vi "Calculadora 1.vi"() -> ()   [LabVIEW 2019]
uses:
  <vilib>/gmath/NI_Gmath.lvlib
panel:
  in  "1/x\nx!":bool
  in  "Ln":bool
  in  "ans":bool
  in  "Pi\ne":bool
  in  "rt^x":bool
  in  "Ship":bool
  in  "e^x":bool
  in  "x^2\nsqrt":bool
  in  "Tanh":bool
  in  "Cosh":bool
  in  "Senh":bool
  in  "Logx":bool
  in  "Tan\nTan^-1":bool
  in  "Cos \nCos^-1":bool
  in  "Sen \nSen^-1":bool
  out "PANTALLA":string
  in  "AC":bool
  in  "C":bool
  in  "+":bool
  in  "=":bool
  in  "0":bool
  in  "/":bool
  in  "9":bool
  in  "8":bool
  in  "7":bool
  in  "X":bool
  in  "6":bool
  in  "5":bool
  in  "4":bool
  in  "-":bool
  in  "3":bool
  in  "2":bool
  in  "1":bool
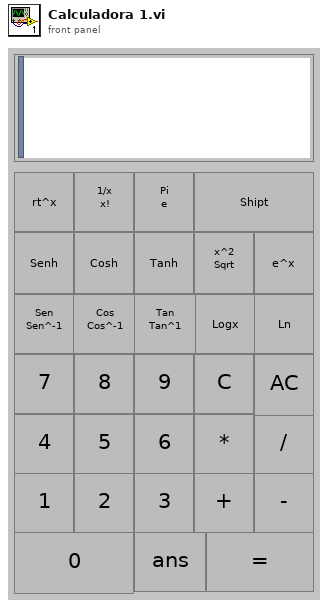
[diagram p1: front panel]
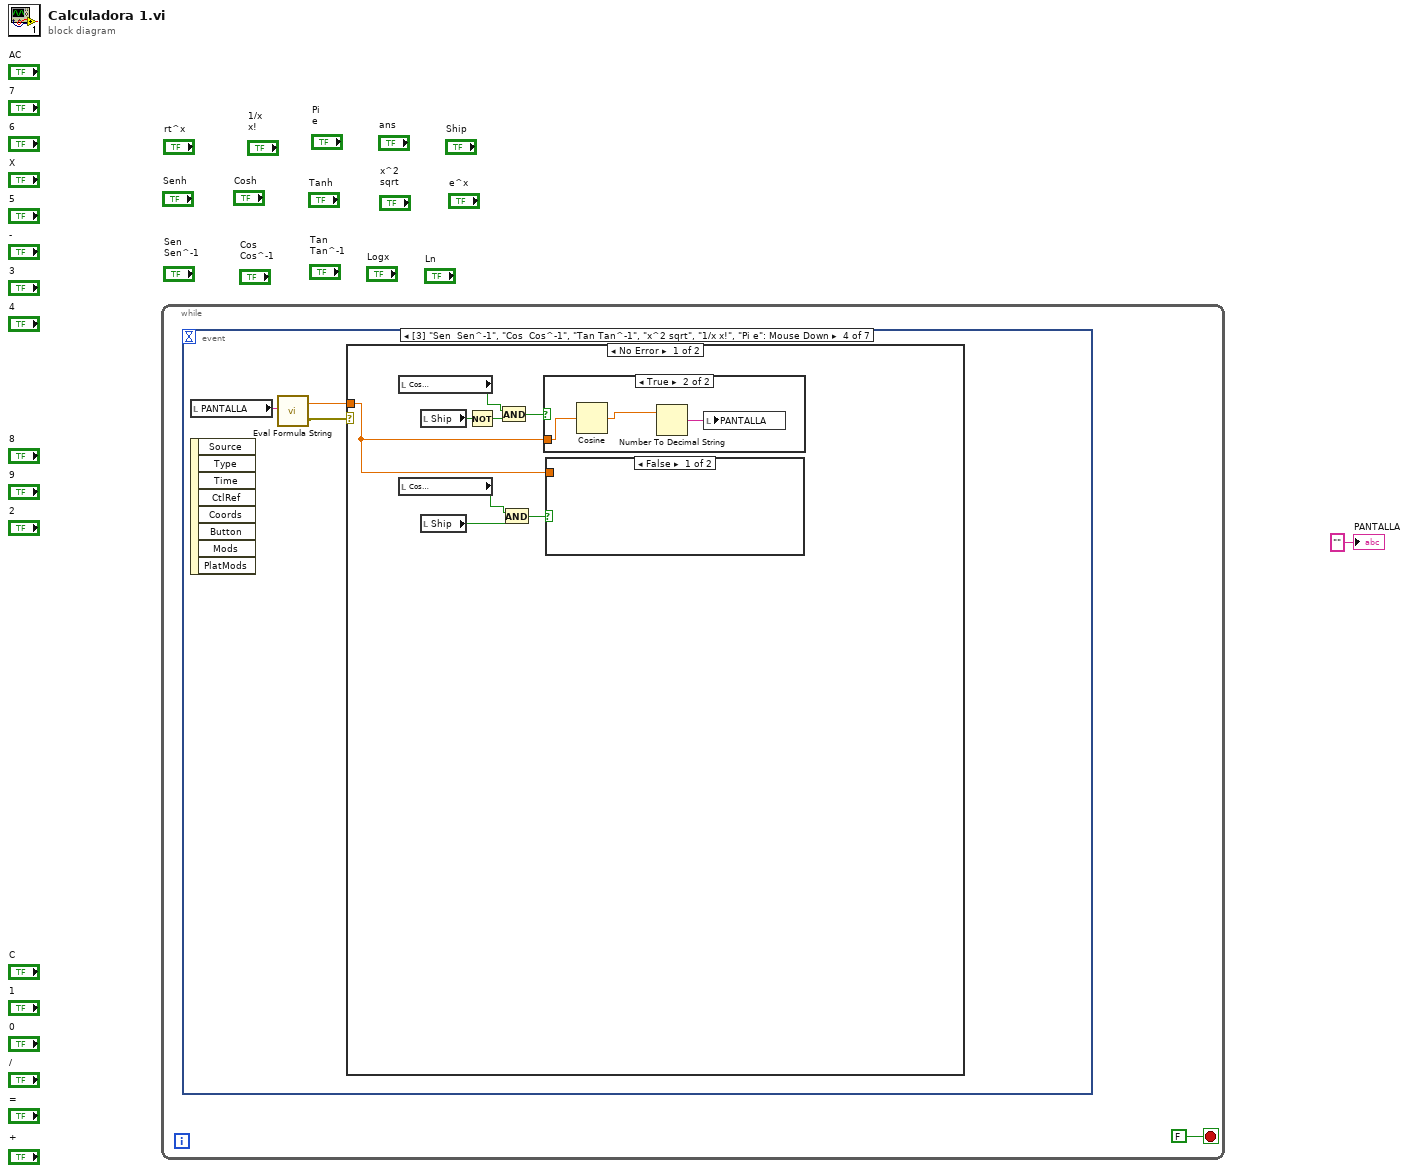
[diagram p0: block diagram]
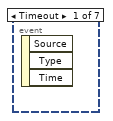
[diagram p2: hidden frame]
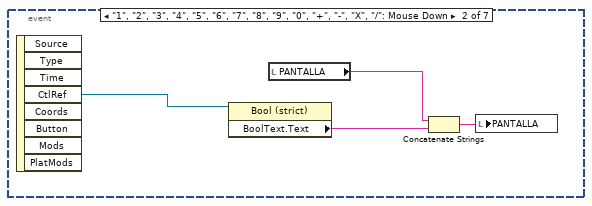
[diagram p3: hidden frame]
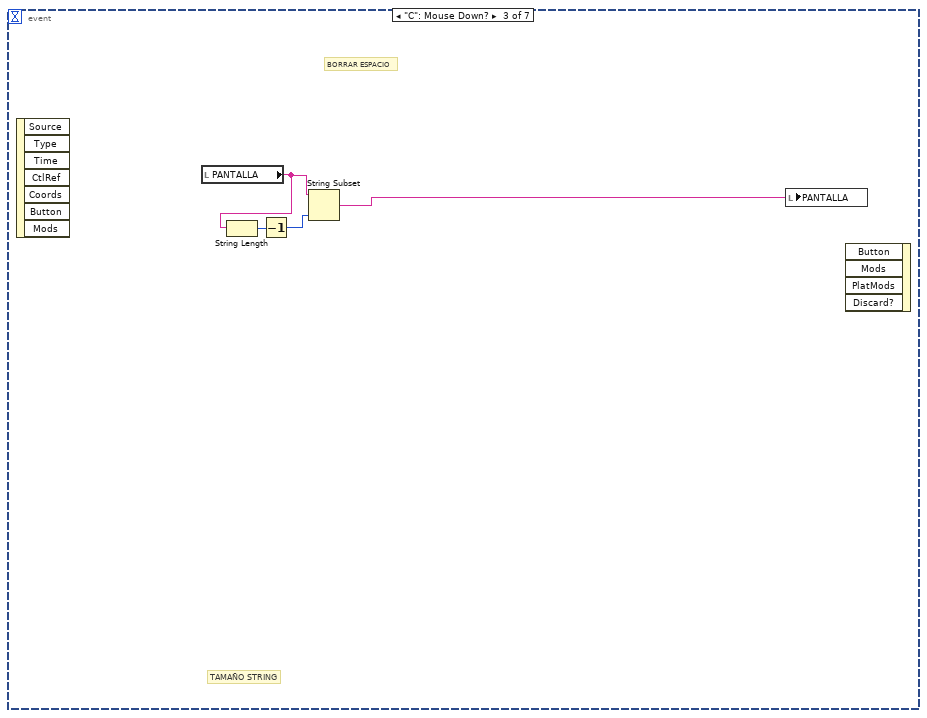
[diagram p4: hidden frame]
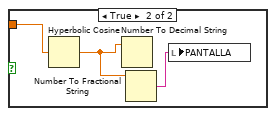
[diagram p6: hidden frame]
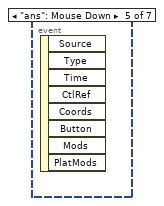
[diagram p8: hidden frame]
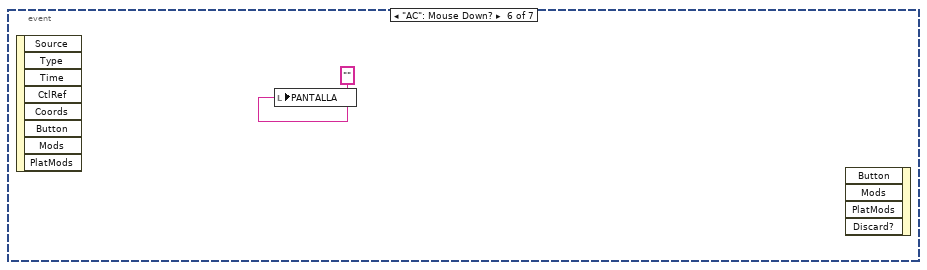
[diagram p9: hidden frame]
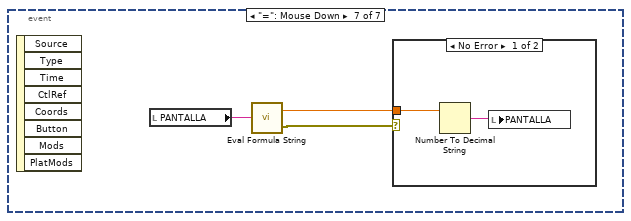
[diagram p10: hidden frame]
diagram:
  n1 = while {
    stop <- FALSE stop-if-true
    n2 = event shown="[3] \"Sen  Sen^-1\", \"Cos  Cos^-1\", \"Tan Tan^-1\", \"x^2 sqrt\", \"1/x x!\", \"Pi e\": Mouse Down" {
      selector: _ -> [_ _ _ _ _ _ _]
      dyn-events: _ -> [_ _ _ _ _ _ _]
      timeout: _ -> [_ _ _ _ _ _ _]
      event Timeout {
        n3 = event-data() -> ()  [unwired: 1 in, 3 out]
      }
      event "1", "2", "3", "4", "5", "6", "7", "8", "9", "0", "+", "-", "X", "/": Mouse Down {
        n4 = event-data() -> ("CtlRef"=w5:refnum<vi>)  [unwired: 1 in, 7 out]
        n5 = property class="Bool (strict)"(reference=w5) -> ("BoolText.Text"=w6:string)  [unwired: 1 in, 2 out]
        n6 = local read "PANTALLA"() -> (w4:string)
        n7 = Concatenate Strings(w4, w6) -> (w3:string)
        n8 = local write "PANTALLA"(w3) -> ()
      }
      event "C": Mouse Down? {
        # "BORRAR ESPACIO"
        # "TAMAÑO STRING"
        n9 = event-data() -> ()  [unwired: 1 in, 7 out]
        n10 = local read "PANTALLA"() -> (w10:string)
        n11 = String Length(string=w10) -> (length=w9:i32)
        n12 = Decrement(x=w9) -> (x-1=w8:i32)
        n13 = String Subset(string=w10, length (rest)=w8) -> (substring=w7:string)  [unwired: 1 in]
        n14 = local write "PANTALLA"(w7) -> ()
        n15 = event-data() -> ()  [unwired: 5 in, 1 out]
      }
      event "Sen \nSen^-1", "Cos \nCos^-1", "Tan\nTan^-1", "x^2\nsqrt", "1/x\nx!", "Pi\ne": Mouse Down {
        n16 = local read "PANTALLA"() -> (w11:string)
        n17 = event-data() -> ()  [unwired: 1 in, 8 out]
        n18 = call <vilib>:"Eval Formula String.vi"("formula"=w11) -> ("error out"=w13:errorcluster, "y value"=w12:dbl)  [unwired: 1 in]
        n19 = case shown="No Error" w13 {
          tunnel: w12 -> [w16 _]
          frame No Error {
            n20 = local read "Cos \nCos^-1"() -> (w18:bool)
            n21 = local read "Cos \nCos^-1"() -> (w19:bool)
            n22 = local read "Ship"() -> (w14:bool)
            n23 = local read "Ship"() -> (w20:bool)
            n24 = Not(x=w14) -> (.not. x?=w15:bool)
            n25 = And(x=w18, y=w15) -> (x .and. y?=w17:bool)
            n26 = And(x=w19, y=w20) -> (x .and. y?=w21:bool)
            n27 = case shown="True" w17 {
              tunnel: w16 -> [_ w24]
              frame False {
              }
              frame True {
                n28 = Cosine(x=w24) -> (cos(x)=w22:dbl)
                n29 = Number To Decimal String(number=w22) -> (decimal integer string=w23:string)  [unwired: 1 in]
                n30 = local write "PANTALLA"(w23) -> ()
              }
            }
            n31 = case shown="False" w21 {
              tunnel: w16 -> [_ w27]
              frame False {
              }
              frame True {
                n32 = Hyperbolic Cosine(1:w27) -> (0:w26:dbl)
                n33 = Number To Decimal String(number=w26) -> ()  [unwired: 1 in, 1 out]
                n34 = Number To Fractional String(number=w26) -> (F-format string=w25:string)  [unwired: 3 in]
                n35 = local write "PANTALLA"(w25) -> ()
              }
            }
          }
          frame Error {
          }
        }
      }
      event "ans": Mouse Down {
        n36 = event-data() -> ()  [unwired: 1 in, 8 out]
      }
      event "AC": Mouse Down? {
        n37 = event-data() -> ()  [unwired: 1 in, 8 out]
        n38 = local write "PANTALLA"("" ("PANTALLA")) -> ()
        n39 = event-data() -> ()  [unwired: 5 in, 1 out]
      }
      event "=": Mouse Down {
        n40 = event-data() -> ()  [unwired: 1 in, 8 out]
        n41 = local read "PANTALLA"() -> (w29:string)
        n42 = call <vilib>:"Eval Formula String.vi"("formula"=w29) -> ("error out"=w31:errorcluster, "y value"=w30:dbl)  [unwired: 1 in]
        n43 = case shown="No Error" w31 {
          tunnel: w30 -> [w33 _]
          frame No Error {
            n44 = Number To Decimal String(number=w33) -> (decimal integer string=w32:string)  [unwired: 1 in]
            n45 = local write "PANTALLA"(w32) -> ()
          }
          frame Error {
          }
        }
      }
    }
  }
  "PANTALLA" <- "" ("PANTALLA")
